vi "Part 2.vi"(11 "Input":string) -> (3 "Output":i64)   [LabVIEW 2021]
uses:
  <userlib>/_OpenG.lib/string/string.llb/Convert EOLs (String)__ogtk.vi
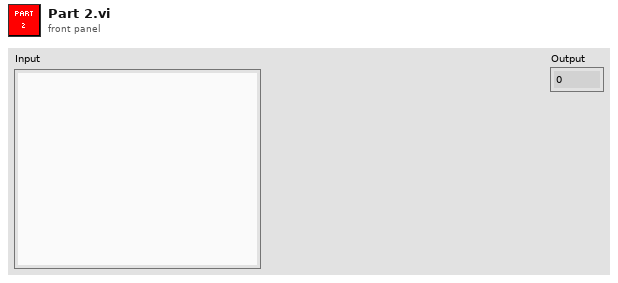
[diagram p1: front panel]
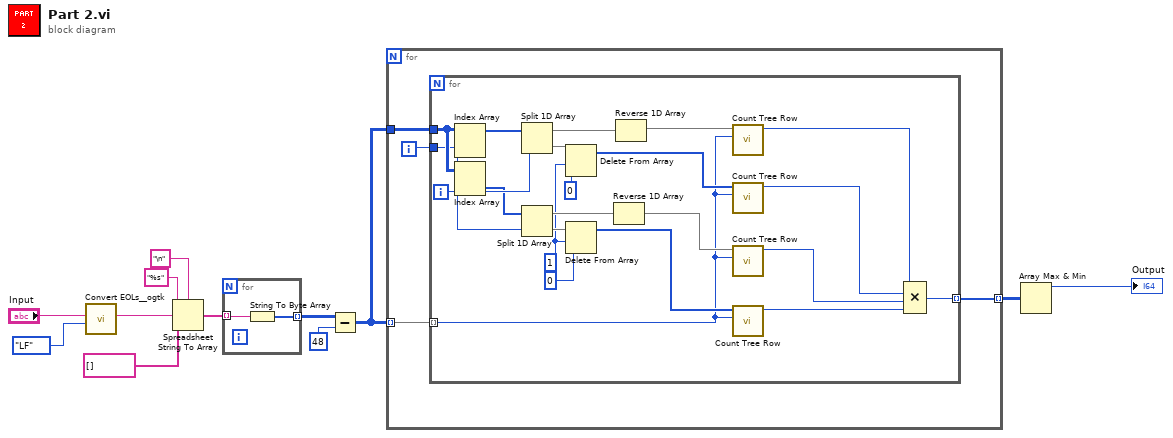
[diagram p0: block diagram]
diagram:
  n1 = call-poly <userlib>:"Convert EOLs__ogtk.vi"("Convert to:"=enum16{"CR", "LF", "CRLF"}."LF", "String in"="Input") -> ("String out"=w9:string)  [unwired: 9 in]
  n2 = Spreadsheet String To Array(delimiter (Tab)="\n", format string="%s", spreadsheet string=w9, array type (2D Dbl)=string[] []) -> (array=w7:string[])
  n3 = for {
    tunnel: w7 -> [w14] mode=indexing
    tunnel: [w13] -> w6 mode=indexing
    n4 = String To Byte Array(string=w14) -> (unsigned byte array=w13:u8[])
  }
  n5 = Subtract(x=w6, y=u8 48) -> (x-y=w4:u8[][])
  n6 = for {
    tunnel: w4 -> [w18] mode=indexing
    tunnel: w4 -> [w17]
    tunnel: [w15] -> w1 mode=indexing
    i -> [w16]
    n7 = for {
      tunnel: w18 -> [w25] mode=indexing
      tunnel: w17 -> [w40]
      tunnel: w16 -> [w36]
      tunnel: [w30] -> w15 mode=indexing
      i -> [w38]
      w20 = 1 ("length")
      n8 = Index Array(array=w40, index (row)=w36) -> (element=w39:u8[])  [unwired: 1 in]
      n9 = Index Array(array=w40, index (col)=w38) -> (element=w37:u8[])  [unwired: 1 in]
      n10 = Split 1D Array(array=w39, index=w38) -> (first subarray=w32:u8[], second subarray=w35:u8[])
      n11 = Split 1D Array(array=w37, index=w36) -> (first subarray=w33:u8[], second subarray=w34:u8[])
      n12 = Delete From Array(array=w35, length=w20, index=0) -> (array with subset deleted=w28:u8[])  [unwired: 1 out]
      n13 = Delete From Array(array=w34, length=w20, index=0) -> (array with subset deleted=w26:u8[])  [unwired: 1 out]
      n14 = Reverse 1D Array(array=w33) -> (reversed array=w27:u8[])
      n15 = Reverse 1D Array(array=w32) -> (reversed array=w29:u8[])
      n16 = call "Count Tree Row.vi"("Tree"=w25, "Tree Row"=w29) -> ("Count"=w23:i64)  [unwired: 9 in]
      n17 = call "Count Tree Row.vi"("Tree"=w25, "Tree Row"=w28) -> ("Count"=w22:i64)  [unwired: 9 in]
      n18 = call "Count Tree Row.vi"("Tree"=w25, "Tree Row"=w27) -> ("Count"=w24:i64)  [unwired: 9 in]
      n19 = call "Count Tree Row.vi"("Tree"=w25, "Tree Row"=w26) -> ("Count"=w21:i64)  [unwired: 9 in]
      n20 = Compound Arithmetic op=MULTIPLY(w23, w22, w24, w21) -> (w30:i64)
    }
  }
  n21 = Array Max & Min(array=w1) -> (max value=→"Output":i64)  [unwired: 3 out]
